vi "Execute.vi"(8 "error in":errorcluster, 11 "SEQ in":refnum<class "SEQ.lvclass">) -> (0 "error out":errorcluster, 1 "Next Step?":bool, 2 "MSG":string, 3 "SEQ out":refnum<class "SEQ.lvclass">)   [LabVIEW 2015, in "Sequence Composition.lvlib" / "SEQ.lvclass"]
doc: "Pop the sequence stack and execute the resulting command on the sequence stack. If the command insists that we need to reinsert the current class, push it back onto the stack. If the message returned by the execution of the step is not empty, load it into the message event queue where it can be handled by the interface."
uses:
  SEQ.lvclass
  SEQ.lvclass/SEQ.ctl
  STEPS/STEP.lvclass
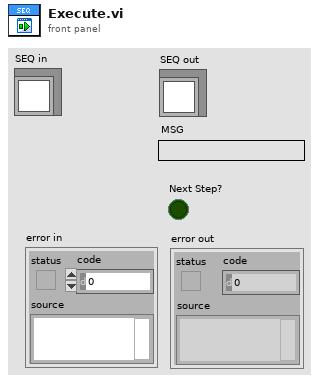
[diagram p1: front panel]
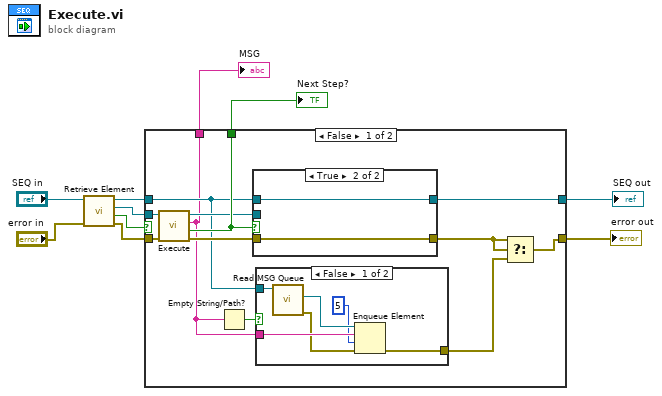
[diagram p0: block diagram]
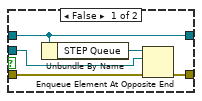
[diagram p3: hidden frame]
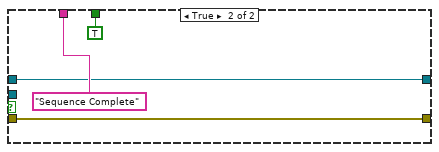
[diagram p4: hidden frame]
diagram:
  n1 = call "Retrieve Element.vi"("error in"="error in", "SEQ in"="SEQ in") -> ("error out"=w6:errorcluster, "empty?"=w1:bool, "STEP.lvclass"=w7:refnum<class "STEP.lvclass">, "SEQ out"=w10:refnum<class "SEQ.lvclass">)  [unwired: 6 in]
  n2 = case shown="False" w1 {
    tunnel: w10 -> [w16 w37]
    tunnel: [w22 w37] -> w9
    tunnel: [w12 w36] -> w8
    tunnel: w7 -> [w20 _]
    tunnel: w6 -> [w19 w36]
    tunnel: [w18 TRUE ("Next Step?")] -> w5
    tunnel: [w14 "Sequence Complete" ("t")] -> w2
    frame False {
      n3 = call-dynamic "Execute.vi"("error in"=w19, "STEP in"=w20) -> ("error out"=w21:errorcluster, "Next Step?"=w18:bool, "MSG"=w14:string, "STEP out"=w17:refnum<class "STEP.lvclass">)  [unwired: 6 in]
      n4 = Empty String/Path?(string/path=w14) -> (empty?=w15:bool)
      n5 = case shown="True" w18 {
        tunnel: w16 -> [w30 w35]
        tunnel: [w30 w35] -> w22
        tunnel: w21 -> [w29 w34]
        tunnel: [w32 w34] -> w13
        tunnel: w17 -> [w31 _]
        frame False {
          n6 = Unbundle By Name(w30) -> ("STEP Queue"=w33:refnum<queue>)
          n7 = Enqueue Element At Opposite End(queue=w33, element=w31, error in (no error)=w29) -> (error out=w32:errorcluster)  [unwired: 1 in, 2 out]
        }
        frame True {
        }
      }
      n8 = case shown="False" w15 {
        tunnel: w16 -> [w27 _]
        tunnel: w14 -> [w28 _]
        tunnel: [w25 _] -> w11
        frame False {
          n9 = call "Read MSG Queue.vi"("SEQ in"=w27) -> ("error out"=w24:errorcluster, "MSG Queue"=w26:refnum<queue>)  [unwired: 8 in, 1 out]
          n10 = Enqueue Element(queue=w26, element=w28, timeout in ms (-1)=5, error in (no error)=w24) -> (error out=w25:errorcluster)  [unwired: 2 out]
        }
        frame True {
        }
      }
      n11 = Select(t=w13, s=w13, f=w11) -> (s? t:f=w12:errorcluster)
    }
    frame True {
    }
  }
  "error out" <- w8
  "SEQ out" <- w9
  "Next Step?" <- w5
  "MSG" <- w2
